vi "addSuccess.vi"(7 "execution time (sec)":dbl, 8 "error in (no error)":errorcluster, 10 "test":refnum<class>, 11 "TestTestResult in":refnum<class "_TextTestResult.JUnitXML.lvclass">) -> (0 "error out":errorcluster, 3 "TestTestResult out":refnum<class "_TextTestResult.JUnitXML.lvclass">)   [LabVIEW 2011, in "_TextTestResult.JUnitXML.lvclass"]
uses:
  _TextTestResult.JUnitXML.lvclass
  <vilib>/addons/_JKI Toolkits/VI Tester/TestResult.llb/resultStatus--enum.ctl
  <vilib>/addons/_JKI Toolkits/VI Tester/_TextTestResult.llb/_TextTestResult.lvclass
  <vilib>/addons/_JKI Toolkits/VI Tester/TestResult.llb/TestResult.lvclass
panel:
  # "JKI VI Tester for LabVIEW\nhttp://jkisoft.com/vi-tester\nCopyright (C) 2007-2009, JKI <info@jkisoft.com>\nALL RIGHTS RESERVED"
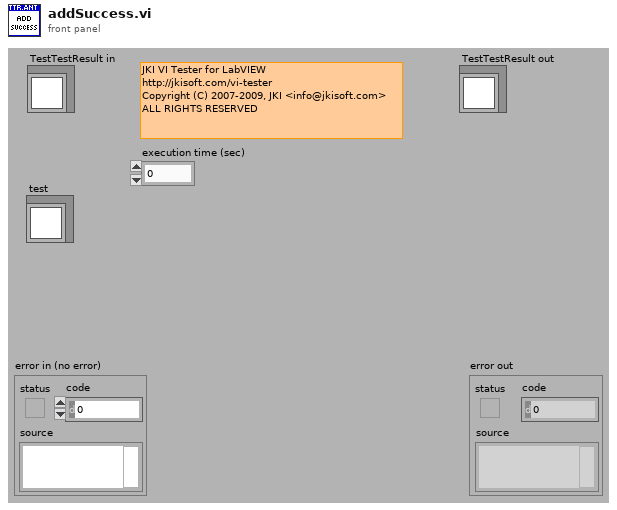
[diagram p1: front panel]
types:
  T1 = typedef "TestResult.lvclass/resultStatus--enum.ctl" = enum16{"testPass", "testFailure", "testError", "testSkipped"}
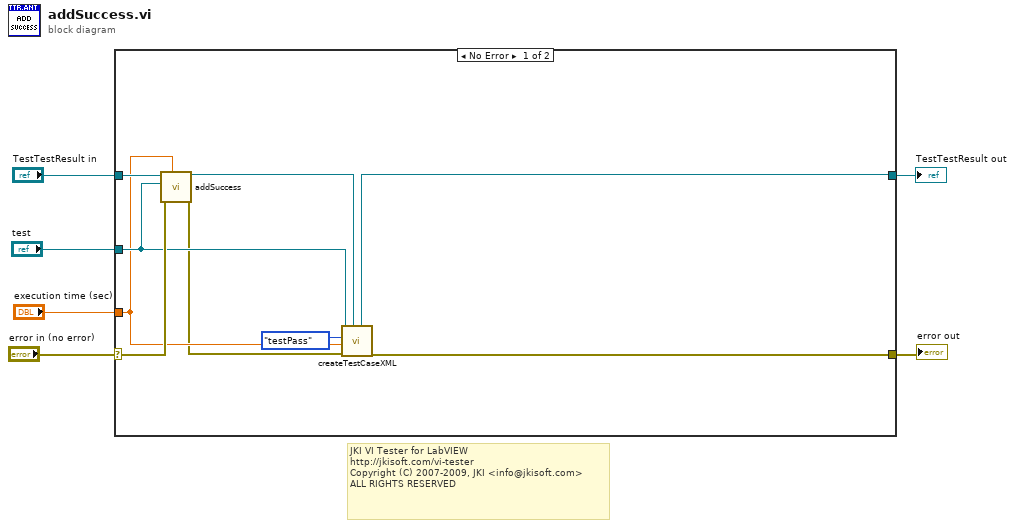
[diagram p0: block diagram]
diagram:
  # "JKI VI Tester for LabVIEW\nhttp://jkisoft.com/vi-tester\nCopyright (C) 2007-2009, JKI <info@jkisoft.com>\nALL RIGHTS RESERVED"
  n1 = case shown="No Error" "error in (no error)" {
    selector: "error in (no error)" -> [w14 w17]
    tunnel: [w9 w17] -> w5
    tunnel: [w7 w16] -> w3
    tunnel: "TestTestResult in" -> [w15 w16]
    tunnel: "test" -> [w12 _]
    tunnel: "execution time (sec)" -> [w11 _]
    frame No Error {
      n2 = call-parent "addSuccess.vi"("execution time (sec)"=w11, "error in (no error)"=w14, "test"=w12, "TestTestResult in"=w15) -> ("error out"=w10:errorcluster, "TestTestResult out"=w8:refnum<class "_TextTestResult.JUnitXML.lvclass">)  [unwired: 6 in]
      n3 = call "createTestCaseXML.vi"("TestTestResult.Ant"=w8, "error in (no error)"=w10, "execution time (sec)"=w11, "resultStatus"=resultStatus--enum."testPass", "Test Out"=w12) -> ("error out"=w9:errorcluster, "TestTestResult.Ant Out"=w7:refnum<class "_TextTestResult.JUnitXML.lvclass">)  [unwired: 5 in]
    }
    frame Error {
    }
  }
  "error out" <- w5
  "TestTestResult out" <- w3
